vi "Set Arm Mode.vi"   [LabVIEW 2013]
uses:
  Robot Global Data.vi
types:
  T1 = enum16{"Hold", "Pick Up", "Catch", "Aim", "Shoot"}[]
  T2 = cluster{"Axes":cluster{"LS X":dbl, "LS Y":dbl, "Triggers":dbl, "RS X":dbl, "RS Y":dbl}, "Buttons":cluster{"LT":bool, "RT":bool, "A":bool, "B":bool, "X":bool, "Y":bool, "LB":bool, "RB":bool, "Back":bool, "Start":bool, "LS":bool, "RS":bool}, "Buttons Just Pushed":cluster{"LT":bool, "RT":bool, "A":bool, "B":bool, "X":bool, "Y":bool, "LB":bool, "RB":bool, "Back":bool, "Start":bool, "LS":bool, "RS":bool}}
  T3 = cluster{"LT":bool, "RT":bool, "A":bool, "B":bool, "X":bool, "Y":bool, "LB":bool, "RB":bool, "Back":bool, "Start":bool, "LS":bool, "RS":bool}
  T4 = enum16{"Hold", "Pick Up", "Catch", "Aim", "Shoot"}
  T5 = typedef "WPI_DigitalInputDevRef.ctl" = cluster{"DevStatus":errorcluster, "DIO Channel":T6, "Digital Module":T7}
  T6 = typedef "FPGA_DIOChannel.ctl" = enum8{"DIO 1", "DIO 2", "DIO 3", "DIO 4", "DIO 5", "DIO 6", "DIO 7", "DIO 8", "DIO 9", "DIO 10", "DIO 11", "DIO 12", "DIO 13", "DIO 14", "Invalid"}
  T7 = typedef "FPGA_TypedefDigitalModule.ctl" = enum16{"Digital Module 1", "Digital Module 2"}
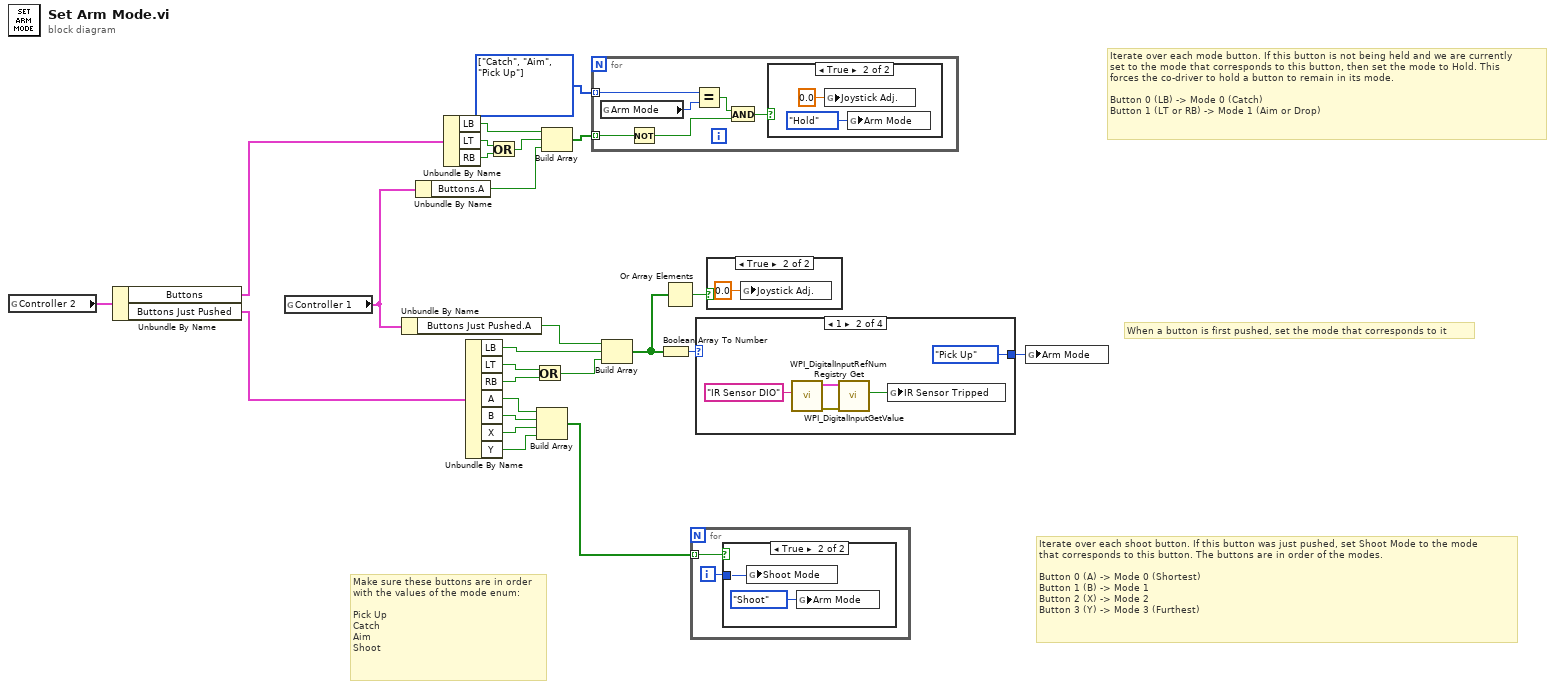
[diagram p0: block diagram]
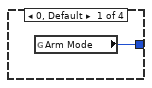
[diagram p3: hidden frame]
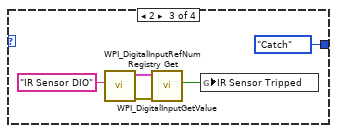
[diagram p4: hidden frame]
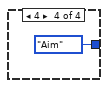
[diagram p5: hidden frame]
diagram:
  w9 = T1 [enum."Catch", enum."Aim", enum."Pick Up"] items=["Hold", "Pick Up", "Catch", "Aim", "Shoot"]
  # "When a button is first pushed, set the mode that corresponds to it"
  # "Iterate over each mode button. If this button is not being held and we are currently\nset to the mode that corresponds to this button, then set the mode to Hold. This\nforces the co-driver to hold a button to remain in its mode.\n\nButton 0 (LB) -> Mode 0 (Catch)\nButton 1 (LT or RB) -> Mode 1 (Aim or Drop)"
  # "Iterate over each shoot button. If this button was just pushed, set Shoot Mode to the mode\nthat corresponds to this button. The buttons are in order of the modes.\n\nButton 0 (A) -> Mode 0 (Shortest)\nButton 1 (B) -> Mode 1\nButton 2 (X) -> Mode 2\nButton 3 (Y) -> Mode 3 (Furthest)"
  # "Make sure these buttons are in order\nwith the values of the mode enum:\n\nPick Up\nCatch\nAim\nShoot"
  n1 = global read "Robot Global Data.vi" "Controller 2"() -> (w15:T2)
  n2 = Unbundle By Name(w15) -> ("Buttons"=w14:T3, "Buttons Just Pushed"=w13:T3)
  n3 = global read "Robot Global Data.vi" "Controller 1"() -> (w2:T2)
  n4 = Unbundle By Name(w2) -> ("Buttons Just Pushed.A"=w3:bool)
  n5 = Unbundle By Name(w2) -> ("Buttons.A"=w1:bool)
  n6 = Unbundle By Name(w14) -> ("LB"=w20:bool, "LT"=w11:bool, "RB"=w12:bool)
  n7 = Unbundle By Name(w13) -> ("LB"=w25:bool, "LT"=w6:bool, "RB"=w5:bool, "A"=w24:bool, "B"=w23:bool, "X"=w22:bool, "Y"=w7:bool)
  n8 = Or(x=w11, y=w12) -> (x .or. y?=w10:bool)
  n9 = Or(x=w6, y=w5) -> (x .or. y?=w4:bool)
  n10 = Build Array(w24, w23, w22, w7) -> (w21:bool[])
  n11 = Build Array(w20, w10, w1) -> (w19:bool[])
  n12 = for {
    tunnel: w19 -> [w29] mode=indexing
    tunnel: w9 -> [w27] mode=indexing
    n13 = global read "Robot Global Data.vi" "Arm Mode"() -> (w26:T4)
    n14 = Not(x=w29) -> (.not. x?=w28:bool)
    n15 = Equal?(x=w27, y=w26) -> (x = y?=w31:bool)
    n16 = And(x=w31, y=w28) -> (x .and. y?=w30:bool)
    n17 = case shown="True" w30 {
      frame False {
      }
      frame True {
        n18 = global write "Robot Global Data.vi" "Joystick Adj."(0.0 ("Joystick Adj.")) -> ()
        n19 = global write "Robot Global Data.vi" "Arm Mode"(T4."Hold" ("Arm Mode")) -> ()
      }
    }
  }
  n20 = Build Array(w3, w25, w4) -> (w16:bool[])
  n21 = Boolean Array To Number(Boolean array=w16) -> (number=w18:u32)
  n22 = Or Array Elements(Boolean array=w16) -> (logical OR=w17:bool)
  n23 = for {
    tunnel: w21 -> [w34] mode=indexing
    i -> [w35]
    n24 = case shown="True" w34 {
      tunnel: w35 -> [_ w37]
      frame False {
      }
      frame True {
        n25 = global write "Robot Global Data.vi" "Shoot Mode"(w37) -> ()
        n26 = global write "Robot Global Data.vi" "Arm Mode"(T4."Shoot" ("Arm Mode")) -> ()
      }
    }
  }
  n27 = case shown="1" w18 {
    tunnel: [w38 T4."Pick Up" ("Arm Mode") T4."Catch" ("Arm Mode") T4."Aim" ("Arm Mode")] -> w8
    frame 0, Default {
      n28 = global read "Robot Global Data.vi" "Arm Mode"() -> (w38:T4)
    }
    frame 1 {
      n29 = call <vilib>:"WPI_DigitalInputRefNum Registry Get.vi"("refnum name"="IR Sensor DIO") -> ("error out"=w42:errorcluster, "DigitalInputDevRef"=w41:T5)  [unwired: 9 in]
      n30 = call <vilib>:"WPI_DigitalInputGetValue.vi"("error in (no error)"=w42, "DigitalInputDevRef"=w41) -> ("Value"=w40:bool)  [unwired: 7 in, 2 out]
      n31 = global write "Robot Global Data.vi" "IR Sensor Tripped"(w40) -> ()
    }
    frame 2 {
      n32 = call <vilib>:"WPI_DigitalInputRefNum Registry Get.vi"("refnum name"="IR Sensor DIO") -> ("error out"=w47:errorcluster, "DigitalInputDevRef"=w46:T5)  [unwired: 9 in]
      n33 = call <vilib>:"WPI_DigitalInputGetValue.vi"("error in (no error)"=w47, "DigitalInputDevRef"=w46) -> ("Value"=w45:bool)  [unwired: 7 in, 2 out]
      n34 = global write "Robot Global Data.vi" "IR Sensor Tripped"(w45) -> ()
    }
    frame 4 {
    }
  }
  n35 = case shown="True" w17 {
    frame False {
    }
    frame True {
      n36 = global write "Robot Global Data.vi" "Joystick Adj."(0.0 ("Joystick Adj.")) -> ()
    }
  }
  n37 = global write "Robot Global Data.vi" "Arm Mode"(w8) -> ()
